vi "SVT Spurious Free Dynamic Range (Time) (1 Ch).vi"(0 "scaled signal [EU]":waveform(dbl)={"t0"=timestamp(0 s since 1904-01-01), "dt"=1e-05, "Y"=[]}, 2 "frequency range":T10={"start frequency"=-1.0, "stop frequency"=-1.0} {"stop frequency" format="%.2f"; "start frequency" format="%.2f"}, 3 "advanced span [Hz]":dbl=-1.0 format="%.2f", 4 "threshold [dBc]":dbl=inf format="%.2f", 5 "error in (no error)":errorcluster, 6 "desired units":T9={"spurious free dynamic range units"=enum."dB", "detected fundamental amplitude units"=enum."EU peak", "dB reference for detected peaks"=enum."dB ref"}, 7 "exclude harmonics":bool, 9 "expected fundamental\nfrequency [Hz]":dbl=-1.0 format="%.2f") -> (11 "detected fundamental\nfrequency [Hz]":dbl=nan format="%.2f", 12 "unit labels":T8, 13 "detected fundamental\namplitude":dbl=nan format="%.2f", 14 "complex spectrum":T7={"complex spectrum response"={"f0"=0.0, "df"=1.0, "complex spectrum"=[]}, "spectrum info"={"channel name"="", "description"="", "x-axis units"=0, "spectral info"={"spectrum type"=enum."Power [Magnitude^2]", "linear/dB"=enum."linear", "window"=0, "window size"=0, "FFT size"=0}, "engineering units"=0, "custom label"="", "dB reference [EU]"=0.0, "peak units"=enum."rms", "weighting filter"=0, "spectral density?"=FALSE, "unit label"="", "spectrum skewed?"=FALSE, "complimentary spectrum units"=enum."none"}} {"spectrum info"."x-axis units" items=["Time (s)"=0, "Frequency-CB (Hz)"=1, "Frequency-CPB (Hz)"=1248, "Frequency-Arbitrary (Hz)"=2357, "Quefrency (s)"=2, "Revolutions (rev)"=3, "Order"=4, "Speed (RPM)"=11, "Speed (rad/s)"=21, "Index"=65535]; "spectrum info"."weighting filter" items=["Linear", "A-weighting", "B-weighting", "C-weighting", "ITU-R 468-4", "Dolby", "CCITT", "C-message", "Wb", "Wc", "Wd", "We", "Wf", "Wh", "Wj", "Wk", "Wm", "AES17 20 kHz lowpass", "AES17 40 kHz lowpass", "AES17 20 kHz highpass", "AES17 40 kHz highpass"]; "spectrum info"."dB reference [EU]" format="%.2f"; "spectrum info"."engineering units" items=["custom..."=0, "V"=1, "A"=21, "C"=30, "pC"=31, "s"=32, "-"=29, "Pa"=2, "N"=20, "g"=3, "m/s^2"=4, "m/s"=5, "m"=6, "mm/s"=12, "mm"=13, "micron/s"=14, "micron"=15, "in/s^2"=7, "in/s"=8, "in"=9, "mil/s"=10, "mil"=11, "rad/s^2"=16, "rad/s"=17, "rad"=18, "deg/s^2"=26, "deg/s"=27, "deg"=28, "RPM"=22, "cycle/s^2"=23, "Hz"=24, "cycle"=25, "strain"=19]; "spectrum info"."spectral info"."window" items=["None "=0, "Hanning"=1, "Hamming"=2, "Blackman-Harris"=3, "Exact Blackman"=4, "Blackman"=5, "Flat Top"=6, "4 Term B-Harris "=7, "7 Term B-Harris"=8, "Low Sidelobe"=9, "Force - Exponential"=10, "Gaussian"=62]; "complex spectrum response"."complex spectrum" format="%.2f"; "complex spectrum response"."df" format="%.2f"; "complex spectrum response"."f0" format="%.2f"}, 16 "spurious free dynamic range":dbl=nan format="%.2f", 17 "detected peaks":cluster{"frequency [Hz]":dbl, "amplitude":dbl}[](array[cluster]) {"amplitude" format="%.2f"; "frequency [Hz]" format="%.2f"}, 18 "index of highest spur":i32, 19 "error out":errorcluster)   [LabVIEW 2017, in "SoundVib_SingleTone.lvlib"]
doc: "Computes the spurious-free dynamic range (SFDR) of <B>scaled signal</B> and returns the detected fundamental frequency, detected fundamental amplitude, spurious free dynamic range, and all detected peaks. Wire data to the <B>scaled signal [EU]</B> input to determine the polymorphic instance to use or manually select the instance."
uses:
  <vilib>/addons/Sound and Vibration/svt_Single Tone Measurements/SoundVib_SingleTone.lvlib
  <vilib>/addons/_NISVFA/_Shared subVIs/Controls/svc_Spectrum Info.ctl
  <vilib>/addons/_NISVFA/_Shared subVIs/Controls/svc_X-Axis Units.ctl
  <vilib>/addons/_NISVFA/_Shared subVIs/Controls/svc_Spectrum Type.ctl
  <vilib>/addons/_NISVFA/_Shared subVIs/Controls/svc_Engineering Units Text Ring.ctl
  <vilib>/addons/_NISVFA/_Shared subVIs/Controls/svc_Weighting Filter Text Ring.ctl
  <vilib>/addons/_NISVFA/_Shared subVIs/Controls/svc_Complimentary Spectrum Units.ctl
  <vilib>/addons/_NISVFA/_Shared subVIs/Controls/svc_Window.ctl
  <vilib>/addons/_NISVFA/_Spectrum Processing/SVFA Spectrum Peak Search.vi
  <vilib>/addons/_NISVFA/_Spectrum Processing/SVFA Spectrum Peak Search (1 Ch).vi
  <vilib>/addons/_NISVFA/_Shared subVIs/Common/svc_Spectrum Units.vi
  <vilib>/addons/_NISVFA/_Spectrum Processing/subVIs/svfa_Spectrum Peak Search.vi
  <vilib>/addons/_NISVFA/_Spectrum Processing/subVIs/svfa_Peak Rough Search Indices.vi
  <vilib>/addons/Sound and Vibration/svt_Distortion/subVIs/sv_Peak View Amplitude (1 Ch).vi
  <vilib>/addons/_NISVFA/_Shared subVIs/Common/svc_Get Weighting Enum and Labels.vi
  <vilib>/addons/_NISVFA/_Shared subVIs/Common/svc_Unit Label Lexical Class.vi
  <vilib>/addons/_NISVFA/_Shared subVIs/Common/svc_Engineering Units to Unit Label.vi
  <vilib>/addons/_NISVFA/_Shared subVIs/Common/svc_Format Value (DBL).vi
  <vilib>/addons/_NISVFA/_Spectrum Processing/subVIs/svfa_Three Finger Peak Search.vi
  <vilib>/Analysis/1siggen.llb/Square Wave.vi
  <vilib>/addons/_NISVFA/_Spectrum Processing/SVFA Unit Conversion.vi
  <vilib>/addons/_NISVFA/_Spectrum Processing/SVFA Unit Conversion (Complex) (1 Ch).vi
  <vilib>/addons/_NISVFA/_Shared subVIs/Common/svc_Check Frequency Range in Spectrum.vi
  <vilib>/addons/_NISVFA/_Shared subVIs/Common/svc_Extract Single Tone Information (complex).vi
  <vilib>/addons/_NISVFA/_Shared subVIs/Common/svc_Window Parameters.vi
  <vilib>/addons/_NISVFA/_Spectrum Processing/SVFA Get Spectrum Subset.vi
  <vilib>/addons/_NISVFA/_Spectrum Processing/SVFA Get Spectrum Subset (Complex) (1 Ch).vi
  <vilib>/addons/Sound and Vibration/svt_Distortion/subVIs/sv_Check Data Valid (Audio) (1 Ch).vi
  <vilib>/addons/Sound and Vibration/svt_Distortion/SoundVib_Distortion.lvlib
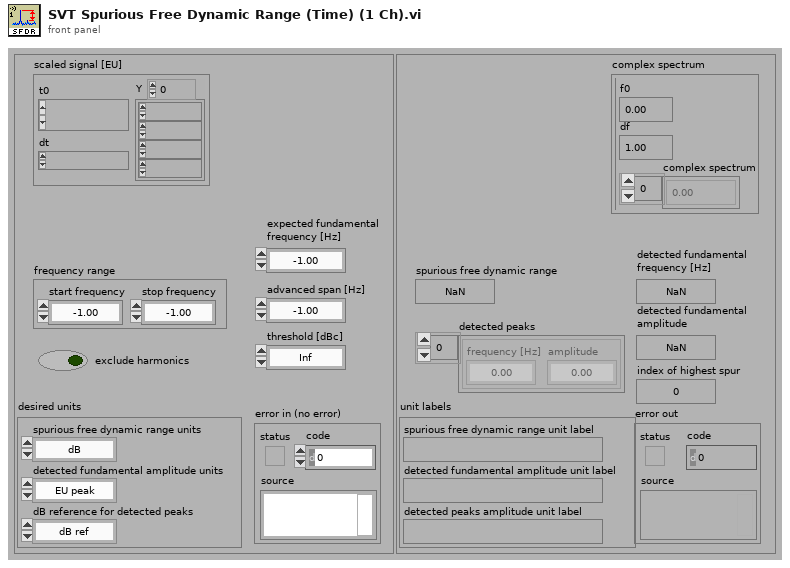
[diagram p1: front panel]
types:
  T1 = typedef "svc_Spectrum Info.ctl" = cluster{"channel name":string, "description":string, "x-axis units":T2, "spectral info":cluster{"spectrum type":T3, "linear/dB":enum16{"linear", "dB"}, "window":u16, "window size":i32, "FFT size":i32}, "engineering units":T4, "custom label":string, "dB reference [EU]":dbl, "peak units":enum16{"rms", "peak", "peak-peak"}, "weighting filter":T5, "spectral density?":bool, "unit label":string, "spectrum skewed?":bool, "complimentary spectrum units":T6}
  T2 = typedef "svc_X-Axis Units.ctl" = u16
  T3 = typedef "svc_Spectrum Type.ctl" = enum16{"FFT Spectrum [complex]", "Amplitude [Magnitude]", "Power [Magnitude^2]", "Cross Spectrum [complex]", "Frequency Response [Complex]"}
  T4 = typedef "svc_Engineering Units Text Ring.ctl" = u16
  T5 = typedef "svc_Weighting Filter Text Ring.ctl" = u16
  T6 = typedef "svc_Complimentary Spectrum Units.ctl" = enum16{"none", "radians", "degrees", "cycles", "imaginary"}
  T7 = cluster{"complex spectrum response":cluster{"f0":dbl, "df":dbl, "complex spectrum":cdb[]}, "spectrum info":T1}
  T8 = cluster{"spurious free dynamic range unit label":string, "detected fundamental amplitude unit label":string, "detected peaks amplitude unit label":string}
  T9 = cluster{"spurious free dynamic range units":enum16{"dB", "ENOB"}, "detected fundamental amplitude units":enum16{"EU rms", "EU peak", "EU peak-peak"}, "dB reference for detected peaks":enum16{"fundamental", "dB ref"}}
  T10 = cluster{"start frequency":dbl, "stop frequency":dbl}
  T11 = cluster{"spurious free dynamic range unit label":string, "detected amplitude unit label":string, "peak amplitude unit label":string}
  T12 = typedef "svc_Window.ctl" = u32
  T13 = cluster{"complex spectrum":cluster{"f0":dbl, "df":dbl, "complex spectrum":cdb[]}, "spectrum info":T1}
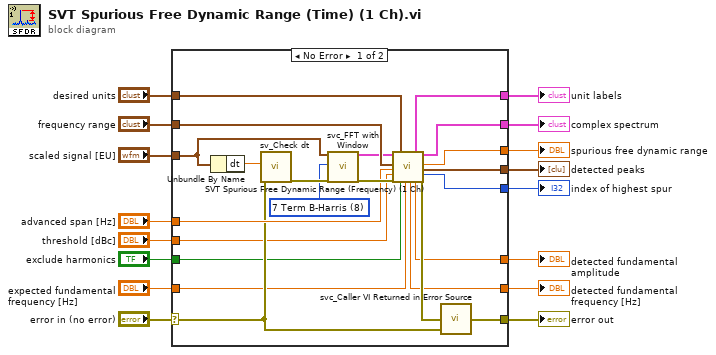
[diagram p0: block diagram]
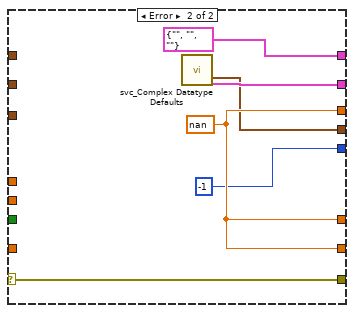
[diagram p2: hidden frame]
diagram:
  n1 = case shown="No Error" "error in (no error)" {
    selector: "error in (no error)" -> [w20 w44]
    tunnel: "scaled signal [EU]" -> [w21 _]
    tunnel: "frequency range" -> [w38 _]
    tunnel: [w34 w42] -> w14
    tunnel: [w27 w44] -> w12
    tunnel: "desired units" -> [w32 _]
    tunnel: [w35 T11 {"spurious free dynamic range unit label"="", "detected amplitude unit label"="", "peak amplitude unit label"=""} ("unit labels")] -> w10
    tunnel: [w31 w40] -> w9
    tunnel: [w30 w39] -> w8
    tunnel: [w28 w42] -> w7
    tunnel: [w29 w42] -> w6
    tunnel: [w25 -1 ("index of highest spur")] -> w5
    tunnel: "advanced span [Hz]" -> [w23 _]
    tunnel: "threshold [dBc]" -> [w19 _]
    tunnel: "exclude harmonics" -> [w18 _]
    tunnel: "expected fundamental\nfrequency [Hz]" -> [w17 _]
    frame No Error {
      w24 = T12 8 items=["None ", "Hanning", "Hamming", "Blackman-Harris", "Exact Blackman", "Blackman", "Flat Top", "4 Term B-Harris ", "7 Term B-Harris", "Low Sidelobe"] ("window")
      n2 = Unbundle By Name(w21) -> ("dt"=w22:dbl)
      n3 = call <vilib>:"sv_Check dt.vi"("error in"=w20, "dt"=w22) -> ("error out"=w26:errorcluster)  [unwired: 8 in, 1 out]
      n4 = call <vilib>:"svc_FFT with Window.vi"("time signal in [EU]"=w21, "window"=w24, "error in (no error)"=w26) -> ("complex spectrum"=w37:T7, "error out"=w36:errorcluster)  [unwired: 15 in]
      n5 = call <vilib>:"SVT Spurious Free Dynamic Range (Frequency) (1 Ch).vi"("complex spectrum"=w37, "frequency range"=w38, "advanced span [Hz]"=w23, "threshold [dBc]"=w19, "error in (no error)"=w36, "desired units"=w32, "exclude harmonics"=w18, "expected fundamental\nfrequency [Hz]"=w17) -> ("detected fundamental\nfrequency [Hz]"=w29:dbl, "unit labels"=w35:T8, "detected fundamental\namplitude"=w28:dbl, "complex spectrum"=w31:T7, "spurious free dynamic range"=w34:dbl, "detected peaks"=w30:cluster{"frequency [Hz]":dbl, "amplitude":dbl}[], "index of highest spur"=w25:i32, "error out"=w33:errorcluster)  [unwired: 4 in]
      n6 = call <vilib>:"svc_Caller VI Returned in Error Source.vi"("warning input to caller"=w20, "error in (no error)"=w33) -> ("error out"=w27:errorcluster)  [unwired: 3 in]
    }
    frame Error {
      w42 = nan
      n7 = call <vilib>:"svc_Complex Datatype Defaults.vi"() -> ("empty array of peaks"=w39:cluster{"frequency":dbl, "value":dbl}[], "complex spectrum"=w40:T13)  [unwired: 11 in, 7 out]
    }
  }
  "spurious free dynamic range" <- w14
  "error out" <- w12
  "complex spectrum" <- w9
  "unit labels" <- w10
  "detected peaks" <- w8
  "detected fundamental\nfrequency [Hz]" <- w6
  "detected fundamental\namplitude" <- w7
  "index of highest spur" <- w5
